vi "Run Ramsete.vi"(7 "Description":string, 8 "Command Info In":T5, 11 "trajectory":T1[](array[typedef])) -> (0 "Command Info Out":T5)   [LabVIEW 2019]
doc: "This VI notifies the subsystem to the new setpoint."
uses:
  <vilib>/Rock Robotics/WPI/Framework/Command Status Info.ctl
  <vilib>/Rock Robotics/WPI/Framework/Completion Status.ctl
  <vilib>/Rock Robotics/WPI/Framework/Completion Notifier.ctl
  Implementation/Drive Setpoints.ctl
  Implementation/Drive Operations.ctl
  <vilib>/Rock Robotics/WPI/ThirdParty/WPILib Extensions/Geometry/Typedef/Translation2d.ctl
  <vilib>/Rock Robotics/WPI/ThirdParty/WPILib Extensions/Geometry/Typedef/Rotation2d.ctl
  <vilib>/Rock Robotics/WPI/ThirdParty/WPILib Extensions/Geometry/Typedef/Pose2d.ctl
  <vilib>/Rock Robotics/WPI/ThirdParty/WPILib Extensions/Trajectory/Typedef/Trajectory State.ctl
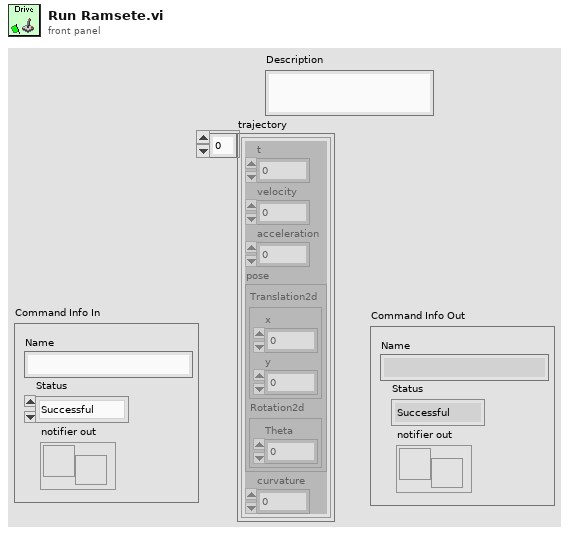
[diagram p1: front panel]
types:
  T1 = typedef "Trajectory State.ctl" = cluster{"t":dbl, "velocity":dbl, "acceleration":dbl, "pose":T2, "curvature":dbl}
  T2 = typedef "Pose2d.ctl" = cluster{"Translation2d":T3, "Rotation2d":T4}
  T3 = typedef "Translation2d.ctl" = cluster{"x":dbl, "y":dbl}
  T4 = typedef "Rotation2d.ctl" = cluster{"Theta":dbl}
  T5 = typedef "Command Status Info.ctl" = cluster{"Name":string, "Status":T6, "notifier out":T7}
  T6 = typedef "Completion Status.ctl" = enum16{"Successful", "Aborted", "Incomplete"}
  T7 = typedef "Completion Notifier.ctl" = refnum<notifier>
  T8 = typedef "Drive Setpoints.ctl" = cluster{"Operation":T9, "Left Setpoint":dbl, "Right Setpoint":dbl, "Duration":dbl, "Data":variant}
  T9 = typedef "Drive Operations.ctl" = enum16{"Reserve", "Read Current", "Immediate", "Drive for Time", "Drive for Distance", "Turn to Angle", "Drivetrain Char", "Pure Pursuit", "Ramsete"}
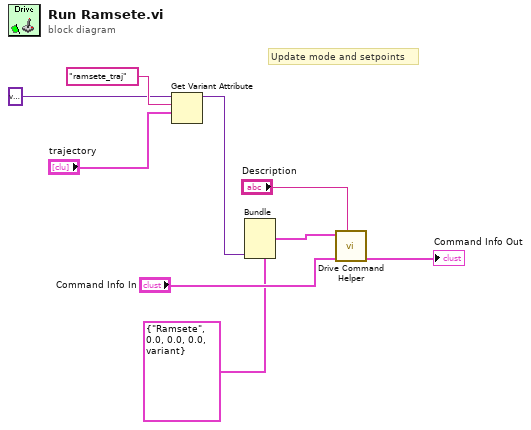
[diagram p0: block diagram]
diagram:
  # "Update mode and setpoints"
  n1 = Get Variant Attribute(Variant=variant ("variant"), name="ramsete_traj", default value (empty Variant)="trajectory") -> (duplicate Variant=w1:variant)  [unwired: 1 in, 3 out]
  n2 = Bundle(cluster=T8 {"Operation"=enum."Ramsete", "Left Setpoint"=0.0, "Right Setpoint"=0.0, "Duration"=0.0, "Data"=variant} ("SubSystem Data"), "Data"=w1) -> (w5:T8)  [unwired: 4 in]
  n3 = call "Drive Command Helper.vi"("Description"="Description", "Command Info In"="Command Info In", "SubSystem Data"=w5) -> ("Command Info Out"=→"Command Info Out":T5)  [unwired: 6 in, 2 out]
